vi "_test_MutatorGAOperator(binary).vi"() -> ()   [LabVIEW 2016]
uses:
  IChromosome/IChromosome.lvclass
  IGene/Children/Binary/_typedefs/BinaryGene_Allele.ctl
  IGene/Children/Binary/Binary Gene.lvclass
  GA Core/Genetic Operators/Mutator/Children/Binary Mutator/Binary Mutator.lvclass
  IGene/Children/RealVal/Real Gene.lvclass
  C:/Users/J51654/My Projects/Evolutionary Programming/GA Framework/IGene/IGene.lvclass
  GA Core/Genetic Operators/Mutator/Children/Real Mutator/Real Mutator.lvclass
  C:/Users/J51654/My Projects/Evolutionary Programming/GA Framework/GA Core/GA Core.lvclass
  GA Core/GA Core.lvclass/GA Core.ctl
  IChromosome/IChromosome.lvclass/IChromosome.ctl
  IGene/Children/RealVal/Real Gene.lvclass/Real Gene.ctl
  IGene/IGene.lvclass
  GA Core/GA Core.lvclass
panel:
  out "After Mutation (R)":dbl[](array[numeric])
  out "Before Mutation (R)":dbl[](array[numeric])
  out "\"matchness\" Real":dbl
  out "\"matchness\"":dbl
  in  "Mutation Rate":dbl=1.0 format="%#_13g"
  out "After Mutation":T1[](array[typedef])
  out "Before Mutation":T1[](array[typedef])
  out "IChromosome out":refnum<class "IChromosome.lvclass">
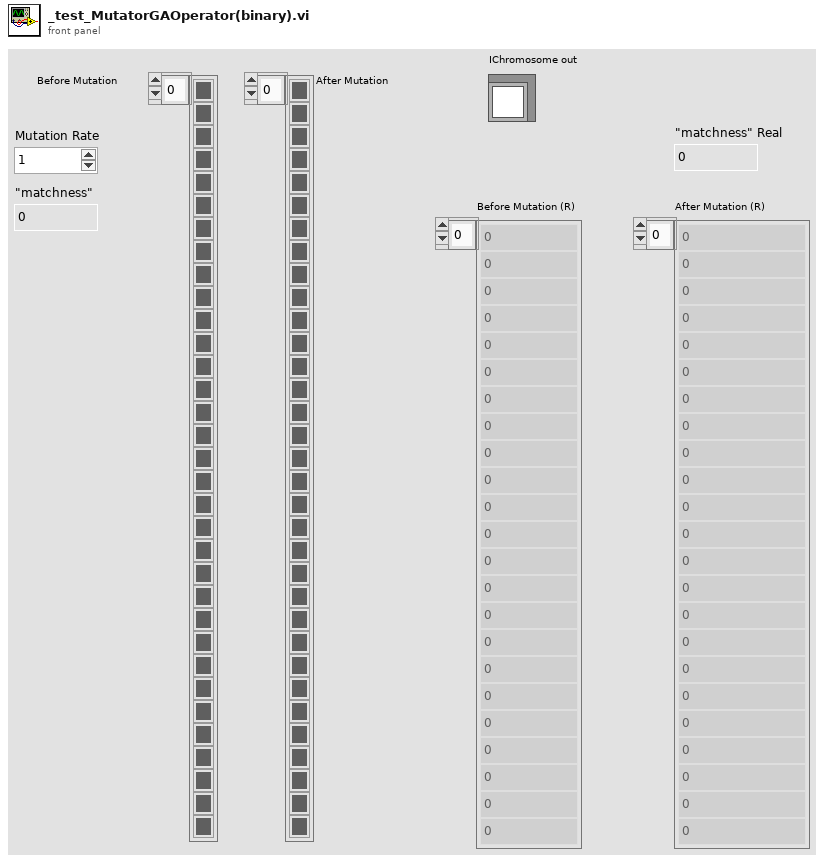
[diagram p1: front panel]
types:
  T1 = typedef "Binary Gene.lvclass/BinaryGene_Allele.ctl" = bool
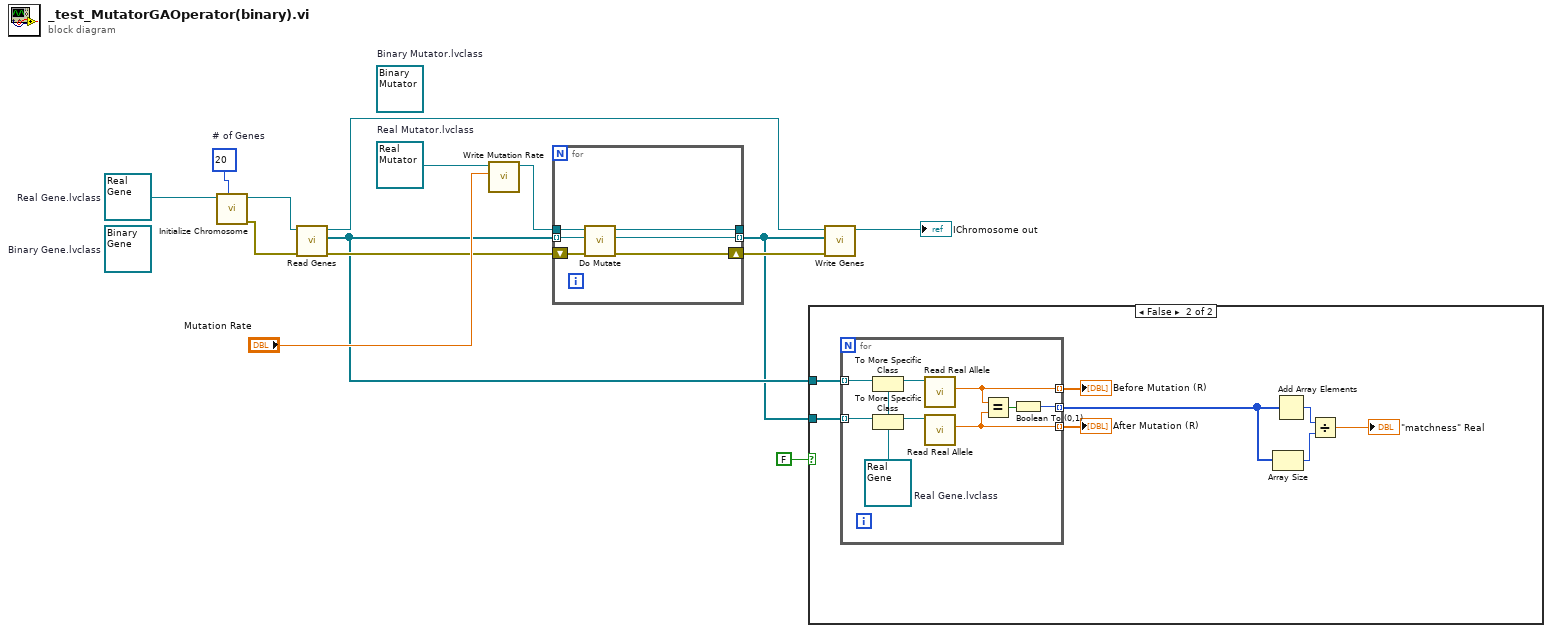
[diagram p0: block diagram]
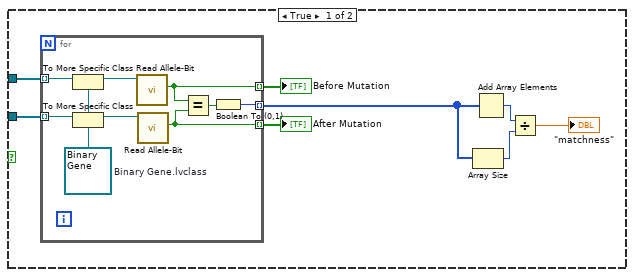
[diagram p2: hidden frame]
diagram:
  w2 = refnum<class "Real Mutator.lvclass"> refnum  # Real Mutator.lvclass
  w3 = refnum<class "Real Gene.lvclass"> refnum  # Real Gene.lvclass
  (unwired) refnum<class "Binary Mutator.lvclass"> refnum  # Binary Mutator.lvclass
  w14 = u32 20  # # of Genes
  (unwired) refnum<class "Binary Gene.lvclass"> refnum  # Binary Gene.lvclass
  n1 = call "Initialize Chromosome.vi"("# of Genes"=w14, "Gene Type In"=w3) -> ("error out"=w6:errorcluster, "Chromosome out"=w13:refnum<class "IChromosome.lvclass">)  [unwired: 8 in]
  n2 = call "Read Genes.vi"("error in (no error)"=w6, "IChromosome in"=w13) -> ("error out"=w9:errorcluster, "Genes"=w5:refnum<class "IGene.lvclass">[], "IChromosome out"=w10:refnum<class "IChromosome.lvclass">)  [unwired: 7 in]
  n3 = call "Write Mutation Rate.vi"("Mutation Rate"="Mutation Rate", "GA Core in"=w2) -> ("GA Core out"=w12:refnum<class "Real Mutator.lvclass">)  [unwired: 8 in, 1 out]
  n4 = for {
    tunnel: w5 -> [w20] mode=indexing
    tunnel: w12 -> [w19]
    tunnel: [w18] -> w4 mode=indexing
    tunnel: [w17] -> _
    shift-right: [w15] -> w8
    shift-left: w9 -> [w16]
    n5 = call-dynamic "Do Mutate.vi"("error in"=w16, "IGene in"=w20, "Real Mutator in"=w19) -> ("error out"=w15:errorcluster, "IGene out"=w18:refnum<class "IGene.lvclass">, "Real Mutator out"=w17:refnum<class "Real Mutator.lvclass">)  [unwired: 6 in]
  }
  n6 = case shown="False" FALSE {
    tunnel: w5 -> [w28 w45]
    tunnel: w4 -> [w27 w44]
    frame True {
      n7 = for {
        tunnel: w28 -> [w37] mode=indexing
        tunnel: w27 -> [w34] mode=indexing
        tunnel: [w32] -> w26 mode=indexing
        tunnel: [w31] -> w25 mode=indexing
        tunnel: [w29] -> w24 mode=indexing
        w35 = refnum<class "Binary Gene.lvclass"> refnum  # Binary Gene.lvclass
        n8 = To More Specific Class(target class=w35, reference=w37) -> (specific class reference=w36:refnum<class "Binary Gene.lvclass">)  [unwired: 1 in, 1 out]
        n9 = To More Specific Class(target class=w35, reference=w34) -> (specific class reference=w33:refnum<class "Binary Gene.lvclass">)  [unwired: 1 in, 1 out]
        n10 = call "Read Allele-Bit.vi"("Binary Gene in"=w36) -> ("Allele-Bit"=w32:T1)  [unwired: 8 in, 2 out]
        n11 = call "Read Allele-Bit.vi"("Binary Gene in"=w33) -> ("Allele-Bit"=w31:T1)  [unwired: 8 in, 2 out]
        n12 = Equal?(x=w32, y=w31) -> (x = y?=w30:T1)
        n13 = Boolean To (0,1)(Boolean=w30) -> (0, 1=w29:i16)
      }
      "Before Mutation" <- w26
      "After Mutation" <- w25
      n14 = Array Size(array=w24) -> (size(s)=w22:i32)
      n15 = Add Array Elements(numeric array=w24) -> (sum=w23:i16)
      n16 = Divide(x=w23, y=w22) -> (x/y=→"\"matchness\"":dbl)
    }
    frame False {
      n17 = for {
        tunnel: w45 -> [w54] mode=indexing
        tunnel: w44 -> [w53] mode=indexing
        tunnel: [w51] -> w43 mode=indexing
        tunnel: [w47] -> w39 mode=indexing
        tunnel: [w46] -> w38 mode=indexing
        w50 = refnum<class "Real Gene.lvclass"> refnum  # Real Gene.lvclass
        n18 = To More Specific Class(target class=w50, reference=w54) -> (specific class reference=w49:refnum<class "Real Gene.lvclass">)  [unwired: 1 in, 1 out]
        n19 = To More Specific Class(target class=w50, reference=w53) -> (specific class reference=w48:refnum<class "Real Gene.lvclass">)  [unwired: 1 in, 1 out]
        n20 = call "Read Real Allele.vi"("Real Gene in"=w49) -> ("Real Allele"=w47:dbl)  [unwired: 8 in, 2 out]
        n21 = call "Read Real Allele.vi"("Real Gene in"=w48) -> ("Real Allele"=w46:dbl)  [unwired: 8 in, 2 out]
        n22 = Equal?(x=w47, y=w46) -> (x = y?=w52:bool)
        n23 = Boolean To (0,1)(Boolean=w52) -> (0, 1=w51:i16)
      }
      "Before Mutation (R)" <- w39
      "After Mutation (R)" <- w38
      n24 = Array Size(array=w43) -> (size(s)=w41:i32)
      n25 = Add Array Elements(numeric array=w43) -> (sum=w42:i16)
      n26 = Divide(x=w42, y=w41) -> (x/y=→"\"matchness\" Real":dbl)
    }
  }
  n27 = call "Write Genes.vi"("error in"=w8, "Genes"=w4, "IChromosome in"=w10) -> ("IChromosome out"=→"IChromosome out":refnum<class "IChromosome.lvclass">)  [unwired: 7 in, 1 out]
